vi "RemoveFromChartCollection.vi"(0 "reference in":refnum<class "LcWebView.lvclass">, 1 "Chart Id":string, 5 "error in (no error)":errorcluster) -> (14 "reference out":refnum<class "LcWebView.lvclass">, 19 "error out":errorcluster)   [LabVIEW 2018, in "LcWebView.lvclass"]
uses:
  LcWebView.lvclass
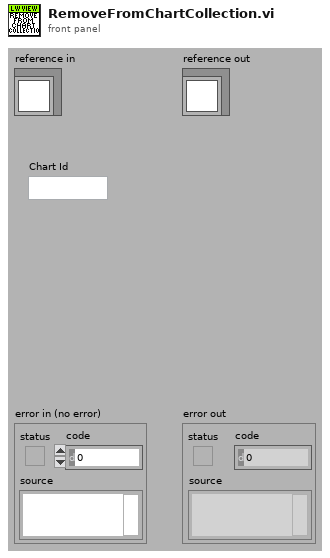
[diagram p1: front panel]
types:
  T1 = typedef "LcWebView.lvclass/ObjectAttributes.ctl" = cluster{"WebView Container":refnum<k24>, "CoreWebViewRef":refnum<k24>, "Status":i32, "Status Message":string, "User Data Folder":path, "BrowserProcessId":u32, "PlotType":T2, "Chart Collection":T3}
  T2 = typedef "LcWebView.lvclass/PlotType.ctl" = enum16{"bar", "line", "pie"}
  T3 = typedef "LcWebView.lvclass/ChartCollection.ctl" = T4[]
  T4 = typedef "LcWebView.lvclass/ChartContent.ctl" = cluster{"Chart Id":string, "Chart Setup":T5, "Chart HTML":string, "Chart Config":string, "Chart Data":string}
  T5 = typedef "LcWebView.lvclass/ChartSetup.ctl" = cluster{"Chart Id":string, "width":u32, "height":u32}
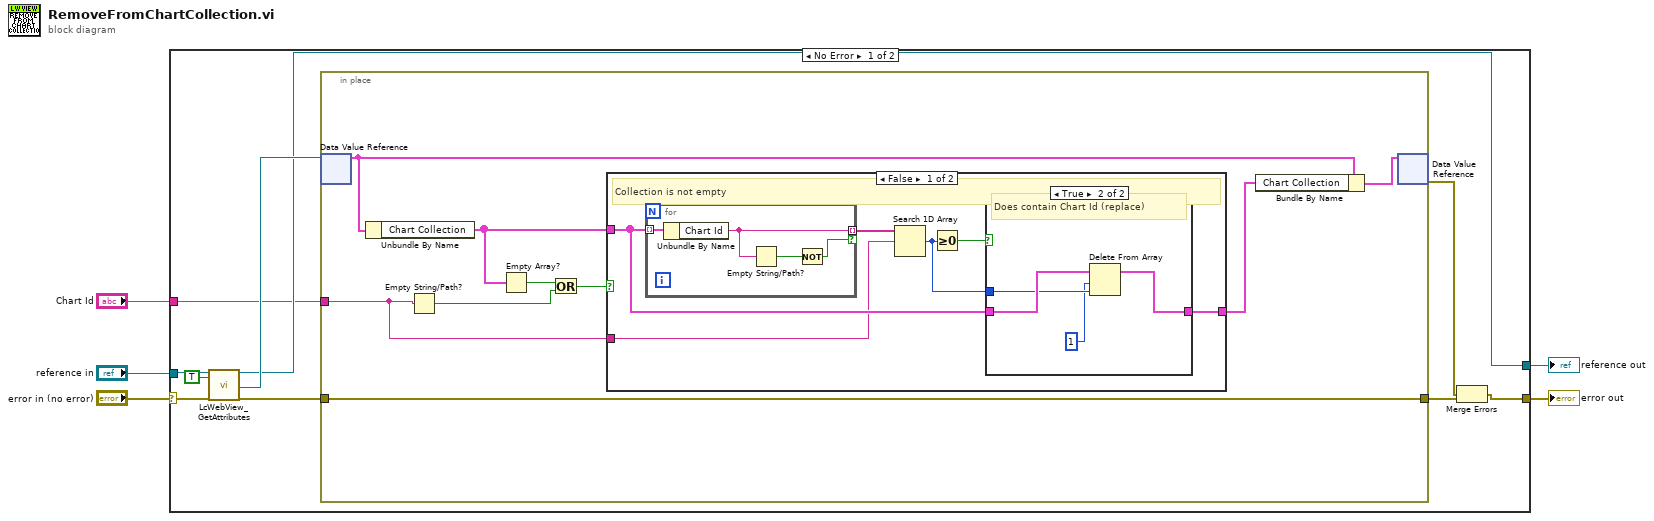
[diagram p0: block diagram]
diagram:
  n1 = case shown="No Error" "error in (no error)" {
    selector: "error in (no error)" -> [w15 w42]
    tunnel: [w7 w42] -> w4
    tunnel: [w10 w41] -> w2
    tunnel: "reference in" -> [w14 w41]
    tunnel: "Chart Id" -> [w6 _]
    frame No Error {
      n2 = call "LcWebView_GetAttributes.vi"("reference in"=w14, "OnlyGetDvrReference(False)"=TRUE, "error in (no error)"=w15) -> ("reference out"=w10:refnum<class "LcWebView.lvclass">, "DataRef"=w13:refnum<data-value>, "error out"=w11:errorcluster)  [unwired: 13 in, 1 out]
      n3 = in-place {
        in-place-border: w11 -> [w20]
        in-place-border: [w20] -> w9
        in-place-border: w6 -> [w16]
        n4 = in-place-dvr #1(w13) -> (w23:T1)  [unwired: 1 out]
        n5 = Unbundle By Name(w23) -> ("Chart Collection"=w24:T3)
        n6 = Empty String/Path?(string/path=w16) -> (empty?=w19:bool)
        n7 = Empty Array?(array=w24) -> (empty?=w18:bool)
        n8 = Or(x=w18, y=w19) -> (x .or. y?=w17:bool)
        n9 = case shown="False" w17 {
          tunnel: w24 -> [w28 w40]
          tunnel: [w27 w40] -> w22
          tunnel: w16 -> [w25 _]
          frame False {
            # "Collection is not empty"
            n10 = for {
              tunnel: w28 -> [w39] mode=indexing
              tunnel: [w38] -> w30 mode=indexing if=w36
              n11 = Unbundle By Name(w39) -> ("Chart Id"=w38:string)
              n12 = Empty String/Path?(string/path=w38) -> (empty?=w37:bool)
              n13 = Not(x=w37) -> (.not. x?=w36:bool)
            }
            n14 = Search 1D Array(1D array=w30, element=w25) -> (index of element=w26:i32)  [unwired: 1 in]
            n15 = Greater Or Equal To 0?(x=w26) -> (x >= 0?=w29:bool)
            n16 = case shown="True" w29 {
              tunnel: w28 -> [w31 w35]
              tunnel: [w31 w32] -> w27
              tunnel: w26 -> [_ w34]
              frame False {
                # "Does not contain (do nothing)"
              }
              frame True {
                # "Does contain Chart Id (replace)"
                n17 = Delete From Array(array=w35, length=1, index=w34) -> (array with subset deleted=w32:T3)  [unwired: 1 out]
              }
            }
          }
          frame True {
            # "Add if collection empty or Chart Id is not valid (do nothing)"
          }
        }
        n18 = Bundle By Name(cluster=w23, "Chart Collection"=w22) -> (w21:T1)
        n19 = in-place-dvr #1(w21) -> (w8:errorcluster)  [unwired: 1 out]
      }
      n20 = Merge Errors(w8, w9) -> (w7:errorcluster)
    }
    frame Error {
    }
  }
  "error out" <- w4
  "reference out" <- w2
